vi "ManipWaitForDistance.vi"(2 "Reinit":bool, 3 "Parameter String":string) -> (0 "Error Out":errorcluster, 1 "Advance Trigger":bool)   [LabVIEW 2023]
doc: "This VI pauses the manipulator sequencer until the robot has driven along a path for a specified distance measured either from the start or the end of the path. It includes an option for a timeout.\n\nParameters:\n1. if postive this is the distance from start of path (in), if negative this is the distance from the end of the path(in)\n2. timeout (ms), or set to -1 to disable"
uses:
  SafeParser_Integer.vi
  SafeParser_Float.vi
  GlobalAutonomous.vi
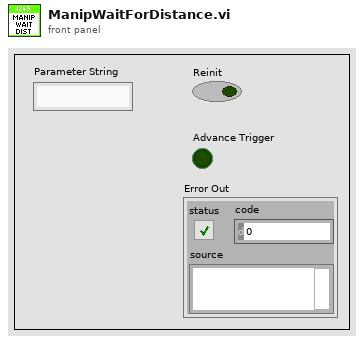
[diagram p1: front panel]
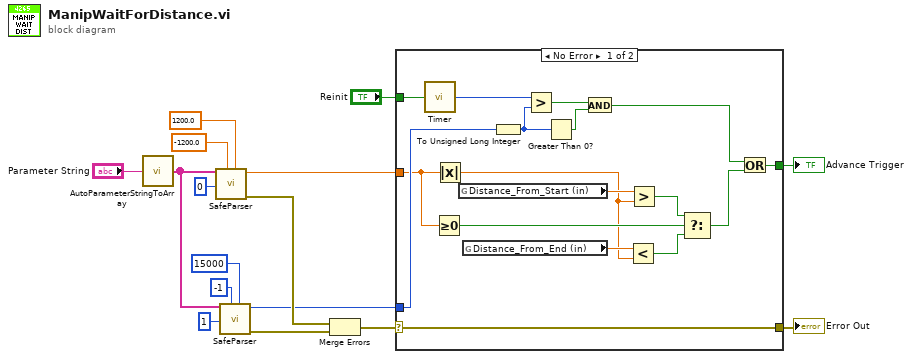
[diagram p0: block diagram]
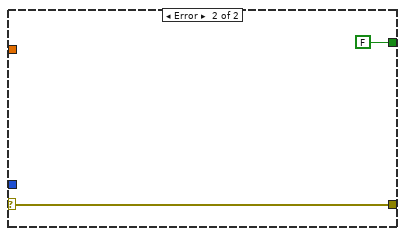
[diagram p2: hidden frame]
diagram:
  n1 = call "AutoParameterStringToArray.vi"("Parameter String"="Parameter String") -> ("Parsed Parameters"=w5:string[])
  n2 = call-poly "SafeParser.vi"("Maximum"=1200.0, "Minimum"=-1200.0, "Array Index"=0 ("Parameter Index"), "String Array"=w5) -> ("Error Out"=w10:errorcluster, "Typecast  Value"=w12:dbl)  [unwired: 6 in]
  n3 = call-poly "SafeParser.vi"("Maximum"=15000, "Minimum"=-1, "Array Index"=1 ("Parameter Index"), "String Array"=w5) -> ("Error Out"=w4:errorcluster, "Typecast  Value"=w3:i32)  [unwired: 6 in]
  n4 = Merge Errors(w10, w4) -> (w9:errorcluster)
  n5 = case shown="No Error" w9 {
    selector: w9 -> [w32 w35]
    tunnel: [w26 FALSE] -> w16
    tunnel: "Reinit" -> [w33 _]
    tunnel: [w32 w35] -> w14
    tunnel: w12 -> [w23 _]
    tunnel: w3 -> [w25 _]
    frame No Error {
      n6 = call "Timer.vi"("Reset Timer"=w33) -> ("Time (ms)"=w28:u32)
      n7 = Greater Or Equal To 0?(x=w23) -> (x >= 0?=w22:bool)
      n8 = Absolute Value(x=w23) -> (abs(x)=w19:dbl)
      n9 = global read "GlobalAutonomous.vi" "Distance_From_Start (in)"() -> (w24:dbl)
      n10 = global read "GlobalAutonomous.vi" "Distance_From_End (in)"() -> (w20:dbl)
      n11 = To Unsigned Long Integer(number=w25) -> (unsigned 32bit integer=w27:u32)
      n12 = Greater?(x=w28, y=w27) -> (0:w31:bool)
      n13 = Greater Than 0?(x=w27) -> (x > 0?=w30:bool)
      n14 = And(x=w31, y=w30) -> (x .and. y?=w29:bool)
      n15 = Less?(x=w20, y=w19) -> (x < y?=w18:bool)
      n16 = Greater?(x=w24, y=w19) -> (0:w21:bool)
      n17 = Select(t=w21, s=w22, f=w18) -> (s? t:f=w17:bool)
      n18 = Or(x=w29, y=w17) -> (x .or. y?=w26:bool)
    }
    frame Error {
    }
  }
  "Advance Trigger" <- w16
  "Error Out" <- w14
